vi "GetInputShapeDim.vi"(7 "DLL path":path, 8 "error in (no error)":errorcluster, 9 "dimIndex":i32, 10 "inputIndex":i32, 11 "session id in":i32) -> (0 "error out":errorcluster, 2 "InputShapeDim":i64, 3 "session id out":i32)   [LabVIEW 2017, in "ONNX Class Library.lvlib"]
doc: "/**\n * @brief Получить значение конкретной размерности входного тензора\n * \n * Возвращает размер тензора по указанному измерению.\n * Например, для shape [1, 3, 224, 224]:\n * - dimIndex=0 вернёт 1 (батч)\n * - dimIndex=1 вернёт 3 (каналы)\n * - dimIndex=2 вернёт 224 (высота)\n * - dimIndex=3 вернёт 224 (ширина)\n * \n * @param sessionId [IN] ID сессии\n * @param inputIndex [IN] Индекс входа (0-based)\n * @param dimIndex [IN] Индекс размерности (0-based, от 0 до GetInputShapeDimCount-1)\n * \n * @return int64: Значение размерности (положительное число)\n * @return int64: -1 если сессия не найдена или индексы неверны\n */\nint64_t GetInputShapeDim(int sessionId, int inputIndex, int dimIndex);"
uses:
  ONNX Class Library.lvlib
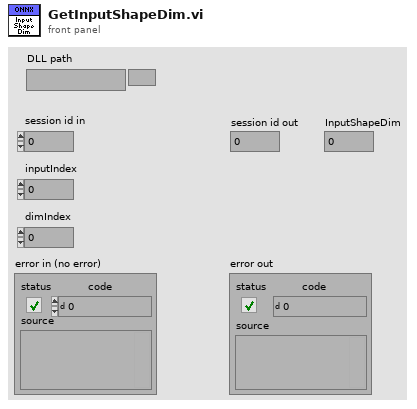
[diagram p1: front panel]
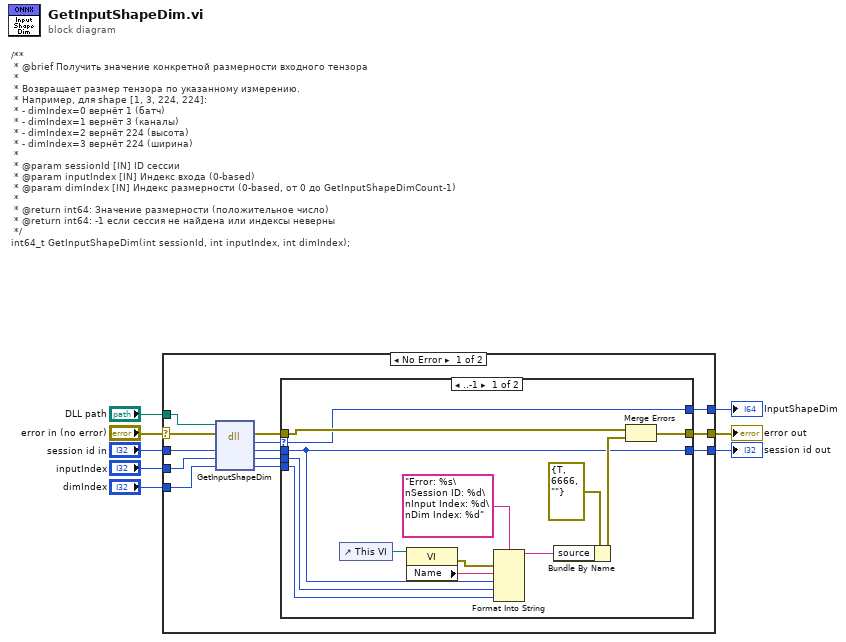
[diagram p0: block diagram]
diagram:
  # "/**\n * @brief Получить значение конкретной размерности входного тензора\n * \n * Возвращает размер тензора по указанному измерению.\n * Например, для shape [1, 3, 224, 224]:\n * - dimIndex=0 вернёт 1 (батч)\n * - dimIndex=1 вернёт 3 (каналы)\n * - dimIndex=2 вернёт 224 (высота)\n * - dimIndex=3 вернёт 224 (ширина)\n * \n * @param sessionId [IN] ID сессии\n * @param inputIndex [IN] Индекс входа (0-based)\n * @param dimIndex [IN] Индекс размерности (0-based, от 0 до GetInputShapeDimCount-1)\n * \n * @return int64: Значение размерности (положительное число)\n * @return int64: -1 если сессия не найдена или индексы неверны\n */\nint64_t GetInputShapeDim(int sessionId, int inputIndex, int dimIndex);"
  n1 = case shown="No Error" "error in (no error)" {
    selector: "error in (no error)" -> [w10 w39]
    tunnel: "inputIndex" -> [w21 _]
    tunnel: "session id in" -> [w20 w38]
    tunnel: "dimIndex" -> [w19 _]
    tunnel: [w15 w39] -> w5
    tunnel: [w14 w38] -> w4
    tunnel: [w13 _] -> w3
    tunnel: "DLL path" -> [w9 _]
    frame No Error {
      n2 = dll-call lib="home/ivan/LabVIEWData/ONNX/Test/libonnx_wrapper/unix64/libonnx_wrapper.so" fn="GetInputShapeDim"(path in=w9, error in=w10, "sessionId"=w20, "inputIndex"=w21, "dimIndex"=w19) -> (error out=w18:errorcluster, "return"=w17:i64, "sessionId"=w16:i32, "inputIndex"=w12:i32, "dimIndex"=w11:i32)  [unwired: 1 in, 1 out]
      n3 = case shown="..-1" w17 {
        selector: w17 -> [w23 w35]
        tunnel: w18 -> [w25 w37]
        tunnel: [w26 w37] -> w15
        tunnel: w16 -> [w27 w36]
        tunnel: [w27 w36] -> w14
        tunnel: w12 -> [w24 _]
        tunnel: [w23 w35] -> w13
        tunnel: w11 -> [w22 _]
        frame ..-1 {
          n4 = control-ref of="This VI"() -> (w31:refnum<vi>)
          n5 = property class="VI"(reference=w31) -> (error out=w28:errorcluster, "Name"=w30:string)  [unwired: 1 in, 1 out]
          n6 = Format Into String(format string="Error: %s\nSession ID: %d\nInput Index: %d\nDim Index: %d", error in=w28, w30, w27, w24, w22) -> (resulting string=w32:string)  [unwired: 1 in, 1 out]
          n7 = Bundle By Name(cluster=errorcluster {"status"=TRUE, "code"=6666, "source"=""} ("error out"), "source"=w32) -> (w33:errorcluster)
          n8 = Merge Errors(w25, w33) -> (w26:errorcluster)
        }
        frame 0.. {
        }
      }
    }
    frame Error {
    }
  }
  "error out" <- w5
  "session id out" <- w4
  "InputShapeDim" <- w3
